vi "Unix Time to Timestamp.vi"(10 "Fractional Second":dbl, 11 "Unix Time (s)":i64) -> (1 "Not a Timestamp?":bool, 3 "Timestamp":timestamp format="%<%H:%M:%S\n%d/%m/%Y>T")   [LabVIEW 2020]
uses:
  Epoch.UNIX.lvclass
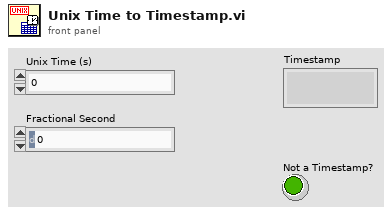
[diagram p1: front panel]
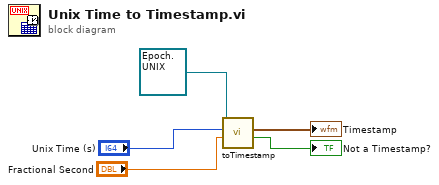
[diagram p0: block diagram]
diagram:
  n1 = call-dynamic "toTimestamp.vi"("Fractional Second"="Fractional Second", "Unix Time (s)"="Unix Time (s)", "Epoch (Unix)"=refnum<class "Epoch.UNIX.lvclass"> refnum ("Epoch.UNIX.lvclass")) -> ("Not a Timestamp?"=→"Not a Timestamp?":bool, "Timestamp"=→"Timestamp":timestamp)  [unwired: 6 in, 1 out]
